vi "global_device_tree_items.vi"() -> ()   [LabVIEW 2015]
panel:
  out "device tree items":T1(array[cluster])=[{"Left Cell String"="NI cRIO (192.168.17.102)", "Child Text"=[], "Child Tag"="NI cRIO", "Item Indent"=0, "Child Only?"=FALSE, "Glyph Index"=1}, {"Left Cell String"="Mod1 (Slot1 NI 9239)", "Child Text"=[], "Child Tag"="Mod1", "Item Indent"=1, "Child Only?"=FALSE, "Glyph Index"=3}, {"Left Cell String"="FCXF-X-02-A01", "Child Text"=[], "Child Tag"="FCXF-X-02-A01", "Item Indent"=2, "Child Only?"=TRUE, "Glyph Index"=4}, {"Left Cell String"="FCXF-X-03-A01", "Child Text"=[], "Child Tag"="FCXF-X-03-A01", "Item Indent"=2, "Child Only?"=TRUE, "Glyph Index"=4}, {"Left Cell String"="FCXF-X-03-A02", "Child Text"=[], "Child Tag"="FCXF-X-03-A02", "Item Indent"=2, "Child Only?"=TRUE, "Glyph Index"=4}, {"Left Cell String"="FCXF-X-04-A01", "Child Text"=[], "Child Tag"="FCXF-X-04-A01", "Item Indent"=2, "Child Only?"=TRUE, "Glyph Index"=4}, {"Left Cell String"="Mod2 (Slot2 NI 9219)", "Child Text"=[], "Child Tag"="Mod2", "Item Indent"=1, "Child Only?"=FALSE, "Glyph Index"=3}, {"Left Cell String"="FCXF-X-02-S01", "Child Text"=[], "Child Tag"="FCXF-X-02-S01", "Item Indent"=2, "Child Only?"=TRUE, "Glyph Index"=4}, {"Left Cell String"="FCXF-X-02-S02", "Child Text"=[], "Child Tag"="FCXF-X-02-S02", "Item Indent"=2, "Child Only?"=TRUE, "Glyph Index"=4}, {"Left Cell String"="FCXF-X-02-S03", "Child Text"=[], "Child Tag"="FCXF-X-02-S03", "Item Indent"=2, "Child Only?"=TRUE, "Glyph Index"=4}, {"Left Cell String"="FCXF-X-02-S04", "Child Text"=[], "Child Tag"="FCXF-X-02-S04", "Item Indent"=2, "Child Only?"=TRUE, "Glyph Index"=4}, {"Left Cell String"="Mod4 (Slot4 NI 9219)", "Child Text"=[], "Child Tag"="Mod4", "Item Indent"=1, "Child Only?"=FALSE, "Glyph Index"=3}, {"Left Cell String"="FCXF-X-03-S01", "Child Text"=[], "Child Tag"="FCXF-X-03-S01", "Item Indent"=2, "Child Only?"=TRUE, "Glyph Index"=4}, {"Left Cell String"="FCXF-X-03-S02", "Child Text"=[], "Child Tag"="FCXF-X-03-S02", "Item Indent"=2, "Child Only?"=TRUE, "Glyph Index"=4}, {"Left Cell String"="FCXF-X-03-S03", "Child Text"=[], "Child Tag"="FCXF-X-03-S03", "Item Indent"=2, "Child Only?"=TRUE, "Glyph Index"=4}, {"Left Cell String"="FCXF-X-03-S04", "Child Text"=[], "Child Tag"="FCXF-X-03-S04", "Item Indent"=2, "Child Only?"=TRUE, "Glyph Index"=4}, {"Left Cell String"="Mod6 (Slot6 NI 9219)", "Child Text"=[], "Child Tag"="Mod6", "Item Indent"=1, "Child Only?"=FALSE, "Glyph Index"=3}, {"Left Cell String"="FCXF-X-03-S05", "Child Text"=[], "Child Tag"="FCXF-X-03-S05", "Item Indent"=2, "Child Only?"=TRUE, "Glyph Index"=4}, {"Left Cell String"="FCXF-X-03-S06", "Child Text"=[], "Child Tag"="FCXF-X-03-S06", "Item Indent"=2, "Child Only?"=TRUE, "Glyph Index"=4}, {"Left Cell String"="Mod8 (Slot8 NI 9219)", "Child Text"=[], "Child Tag"="Mod8", "Item Indent"=1, "Child Only?"=FALSE, "Glyph Index"=3}, {"Left Cell String"="FCXF-X-04-S01", "Child Text"=[], "Child Tag"="FCXF-X-04-S01", "Item Indent"=2, "Child Only?"=TRUE, "Glyph Index"=4}, {"Left Cell String"="FCXF-X-04-S02", "Child Text"=[], "Child Tag"="FCXF-X-04-S02", "Item Indent"=2, "Child Only?"=TRUE, "Glyph Index"=4}, {"Left Cell String"="FCXF-X-04-S03", "Child Text"=[], "Child Tag"="FCXF-X-04-S03", "Item Indent"=2, "Child Only?"=TRUE, "Glyph Index"=4}, {"Left Cell String"="FCXF-X-04-S04", "Child Text"=[], "Child Tag"="FCXF-X-04-S04", "Item Indent"=2, "Child Only?"=TRUE, "Glyph Index"=4}, {"Left Cell String"="Mod9 (USB1 ICPCON 7005)", "Child Text"=[], "Child Tag"="Mod9", "Item Indent"=1, "Child Only?"=FALSE, "Glyph Index"=3}, {"Left Cell String"="FCXF-X-02-T01", "Child Text"=[], "Child Tag"="FCXF-X-02-T01", "Item Indent"=2, "Child Only?"=TRUE, "Glyph Index"=4}, {"Left Cell String"="FCXF-X-02-T02", "Child Text"=[], "Child Tag"="FCXF-X-02-T02", "Item Indent"=2, "Child Only?"=TRUE, "Glyph Index"=4}, {"Left Cell String"="FCXF-X-02-T03", "Child Text"=[], "Child Tag"="FCXF-X-02-T03", "Item Indent"=2, "Child Only?"=TRUE, "Glyph Index"=4}, {"Left Cell String"="FCXF-X-02-T04", "Child Text"=[], "Child Tag"="FCXF-X-02-T04", "Item Indent"=2, "Child Only?"=TRUE, "Glyph Index"=4}, {"Left Cell String"="FCXF-X-03-T01", "Child Text"=[], "Child Tag"="FCXF-X-03-T01", "Item Indent"=2, "Child Only?"=TRUE, "Glyph Index"=4}, {"Left Cell String"="FCXF-X-03-T02", "Child Text"=[], "Child Tag"="FCXF-X-03-T02", "Item Indent"=2, "Child Only?"=TRUE, "Glyph Index"=4}, {"Left Cell String"="FCXF-X-03-T03", "Child Text"=[], "Child Tag"="FCXF-X-03-T03", "Item Indent"=2, "Child Only?"=TRUE, "Glyph Index"=4}, {"Left Cell String"="Mod10 (USB1 ICPCON 7005)", "Child Text"=[], "Child Tag"="Mod10", "Item Indent"=1, "Child Only?"=FALSE, "Glyph Index"=3}, {"Left Cell String"="FCXF-X-03-T04", "Child Text"=[], "Child Tag"="FCXF-X-03-T04", "Item Indent"=2, "Child Only?"=TRUE, "Glyph Index"=4}, {"Left Cell String"="FCXF-X-03-T05", "Child Text"=[], "Child Tag"="FCXF-X-03-T05", "Item Indent"=2, "Child Only?"=TRUE, "Glyph Index"=4}, {"Left Cell String"="FCXF-X-03-T06", "Child Text"=[], "Child Tag"="FCXF-X-03-T06", "Item Indent"=2, "Child Only?"=TRUE, "Glyph Index"=4}, {"Left Cell String"="FCXF-X-04-T01", "Child Text"=[], "Child Tag"="FCXF-X-04-T01", "Item Indent"=2, "Child Only?"=TRUE, "Glyph Index"=4}, {"Left Cell String"="FCXF-X-04-T02", "Child Text"=[], "Child Tag"="FCXF-X-04-T02", "Item Indent"=2, "Child Only?"=TRUE, "Glyph Index"=4}, {"Left Cell String"="FCXF-X-04-T03", "Child Text"=[], "Child Tag"="FCXF-X-04-T03", "Item Indent"=2, "Child Only?"=TRUE, "Glyph Index"=4}, {"Left Cell String"="FCXF-X-04-T04", "Child Text"=[], "Child Tag"="FCXF-X-04-T04", "Item Indent"=2, "Child Only?"=TRUE, "Glyph Index"=4}] caption="设备树项目"
  # "在Utility - Edit Device Tree Items.vi 中编辑树形控件并执行生成config.txt，将配置文件拷贝至控制器c文件夹。实时应用运行时将自动更新该全局变量。"
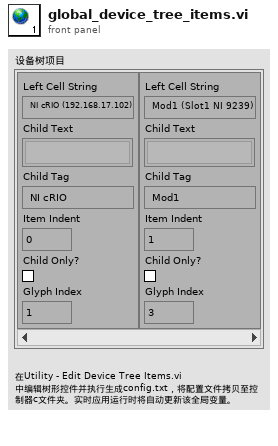
[diagram p1: front panel]
types:
  T1 = cluster{"Left Cell String":string, "Child Text":string[], "Child Tag":string, "Item Indent":i32, "Child Only?":bool, "Glyph Index":i32}[]
diagram:
